vi "Event Handler.vi"(0 "uService Template in":refnum<class "Pizza Machine.lvclass">, 5 "Event type":T1=enum."Message", 7 "Item Name":string, 9 "Data":variant, 11 "error in (no error)":errorcluster) -> (4 "uService Template out":refnum<class "Pizza Machine.lvclass">, 15 "error out":errorcluster)   [LabVIEW 2020, in "Pizza Machine.lvlib" / "Pizza Machine.lvclass"]
doc: "This VI is the event handler of the uService: every time an event is triggered to the uService, this VI is called.\nNote: here you can access the Actor/Class data, but it will be the one coming out from Init. You cannot modify the values.\nThree different events are supported:\nI) Button Pressed: get called on a GUI button pressed. Item Name is the name (label) of the button, Data is empty.\nII) Shared Variable Updated: get called when a SV you subscribed to is updated. Item Name is the name of the SV, and Data is the value (note: you need to convert it to the proper type).\nIII) Message: get called every time a user event is generated using Send Message to Event Handler. The values of Item Name and Data are the one given to the Send Message to Event Handler.\nIV) Ready to launch?: this frame get called every time a new Run is initiated. Each uService is responsible of performing a self check before giving back the green light for the Run to start."
uses:
  Pizza Machine.lvclass
  TALOS/TALOS_PPL.lvlibp/Father of all uServices/Father of all uServices/Event Handler Items.ctl
  Pizza Machine Consumer Case Selector.ctl
  TALOS/TALOS_PPL.lvlibp/Father of all uServices/Father of all uServices/Father of all uServices.lvclass
  Pizza Machine.lvclass/Pizza Machine.ctl
  TALOS/TALOS_PPL.lvlibp
  C:/LabVIEW Code/aegis-labview-code/TALOS/TALOS_PPL.lvlibp/Father of all uServices/Father of all uServices/Father of all uServices.lvclass
  C:/LabVIEW Code/aegis-labview-code/TALOS/TALOS_PPL.lvlibp/Ancestor/Ancestor/Ancestor.lvclass
  C:/LabVIEW Code/aegis-labview-code/TALOS/Actor Framework.lvlibp/1abvi3w/vi.lib/ActorFramework/Actor/Actor.lvclass
  C:/LabVIEW Code/aegis-labview-code/Other uServices/Pizza Machine/Pizza Machine.lvclass
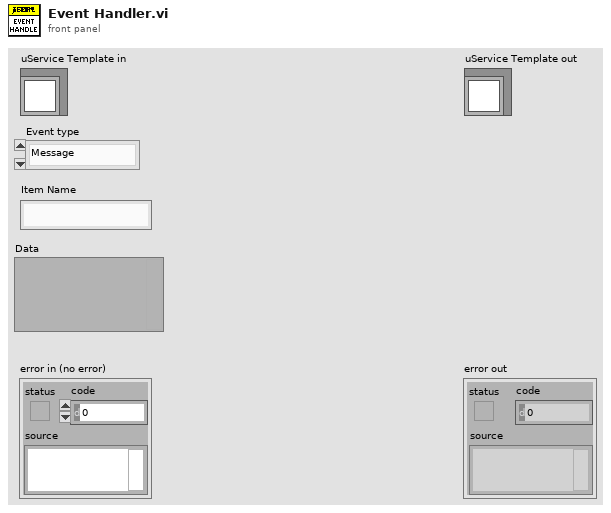
[diagram p1: front panel]
types:
  T1 = typedef "TALOS_PPL.lvlibp/Father of all uServices.lvlib/Father of all uServices.lvclass/Event Handler Items.ctl" = enum16{"Button Pressed", "Shared Variable Updated", "Message", "Ready to launch?", "Safe Mode", "Start RUN", "Stop RUN"}
  T2 = typedef "Pizza Machine.lvlib/Pizza Machine.lvclass/Pizza Machine Consumer Case Selector.ctl" = enum16{"Make Pizza"}
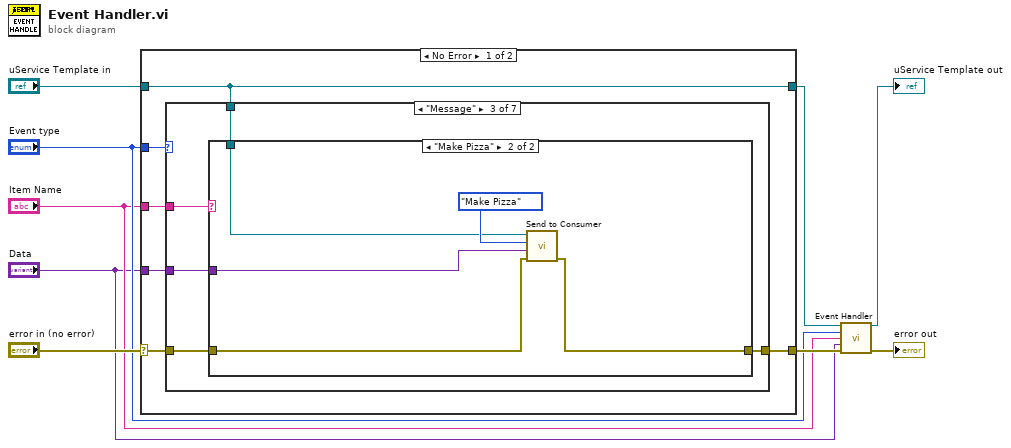
[diagram p0: block diagram]
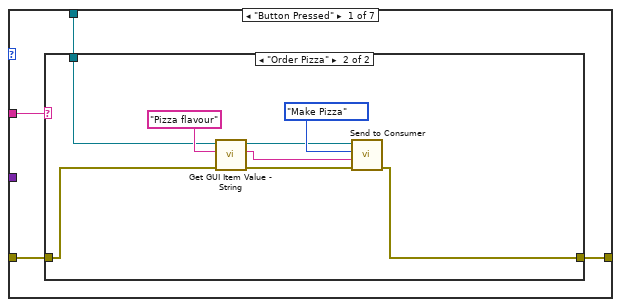
[diagram p2: hidden frame]
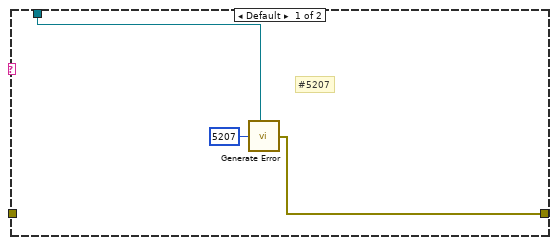
[diagram p3: hidden frame]
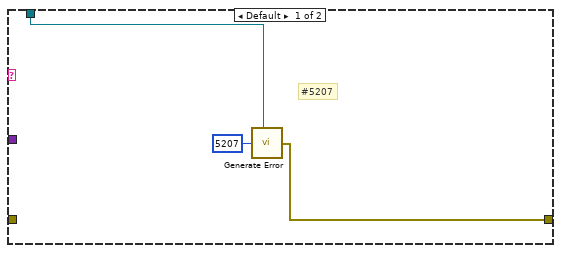
[diagram p5: hidden frame]
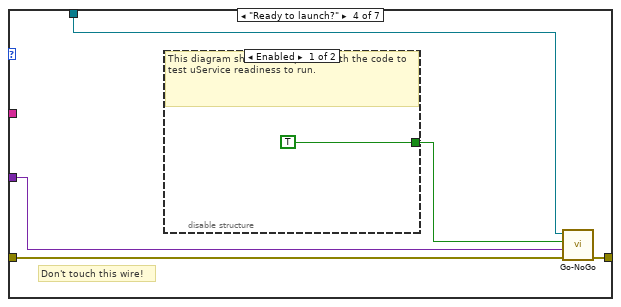
[diagram p6: hidden frame]
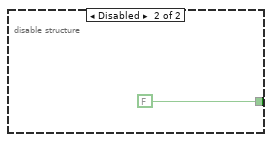
[diagram p7: hidden frame]
diagram:
  n1 = case shown="No Error" "error in (no error)" {
    selector: "error in (no error)" -> [w13 w56]
    tunnel: [w14 w56] -> w7
    tunnel: [w12 w55] -> w4
    tunnel: "uService Template in" -> [w12 w55]
    tunnel: "Event type" -> [w15 _]
    tunnel: "Item Name" -> [w11 _]
    tunnel: "Data" -> [w10 _]
    frame No Error {
      n2 = case shown="\"Message\"" w15 {
        tunnel: [w19 w31 w32 w48 w52 w53 w54] -> w14
        tunnel: w13 -> [w16 w31 w36 w49 w52 w53 w54]
        tunnel: w11 -> [w17 _ w35 _ _ _ _]
        tunnel: w12 -> [w18 _ w33 w47 _ _ _]
        tunnel: w10 -> [_ _ w34 w45 _ _ _]
        frame "Button Pressed" {
          n3 = case shown="\"Order Pizza\"" w17 {
            tunnel: w16 -> [_ w24]
            tunnel: [w20 w29] -> w19
            tunnel: w18 -> [w21 w27]
            frame Default {
              # "#5207"
              n4 = call "Generate Error.vi"("Class"=w21, "Error Code"=5207) -> ("error out"=w20:errorcluster)  [unwired: 5 in]
            }
            frame "Order Pizza" {
              n5 = call "Get GUI Item Value - String.vi"("error in (no error)"=w24, "FP Item Name"="Pizza flavour", "uService Template in"=w27) -> ("error out"=w23:errorcluster, "Value"=w25:string, "uService Template out"=w26:refnum<class "Pizza Machine.lvclass">)  [unwired: 6 in]
              n6 = call "Send to Consumer.vi"("error in (no error)"=w23, "Data"=w25, "Case ID"=Pizza_Machine_Consumer_Case_Selector."Make Pizza" ("Consumer Case Selector"), "uService Template in"=w26) -> ("error out"=w29:errorcluster)  [unwired: 6 in, 1 out]
            }
          }
        }
        frame "Shared Variable Updated" {
        }
        frame "Message" {
          n7 = case shown="\"Make Pizza\"" w35 {
            tunnel: w36 -> [_ w40]
            tunnel: w34 -> [_ w42]
            tunnel: w33 -> [w38 w43]
            tunnel: [w37 w41] -> w32
            frame Default {
              # "#5207"
              n8 = call "Generate Error.vi"("Class"=w38, "Error Code"=5207) -> ("error out"=w37:errorcluster)  [unwired: 5 in]
            }
            frame "Make Pizza" {
              n9 = call "Send to Consumer.vi"("error in (no error)"=w40, "Data"=w42, "Case ID"=Pizza_Machine_Consumer_Case_Selector."Make Pizza" ("Consumer Case Selector"), "uService Template in"=w43) -> ("error out"=w41:errorcluster)  [unwired: 6 in, 1 out]
            }
          }
        }
        frame "Ready to launch?" {
          # "Don't touch this wire!"
          n10 = disable-structure shown="Enabled" {
            disable-tunnel: [TRUE ("Go?") FALSE ("Go?")] -> w46
            frame Enabled {
              # "This diagram should be replaced with the code to test uService readiness to run."
            }
            frame Disabled {
            }
          }
          n11 = call-dynamic "Go-NoGo.vi"("error in (no error)"=w49, "Go-NoGo Data"=w45, "Go?"=w46, "Father of all uServices in"=w47) -> ("error out"=w48:errorcluster)  [unwired: 6 in, 1 out]
        }
        frame "Safe Mode" {
          # "This case gets triggered"
        }
        frame "Start RUN" {
        }
        frame "Stop RUN" {
        }
      }
    }
    frame Error {
    }
  }
  n12 = call-parent "Event Handler.vi"("uService Template in"=w4, "Event type"="Event type", "Item Name"="Item Name", "Data"="Data", "error in (no error)"=w7) -> ("uService Template out"=→"uService Template out":refnum<class "Pizza Machine.lvclass">, "error out"=→"error out":errorcluster)  [unwired: 9 in]
